vi "Noise Cancel.vi"(9 "Config":T2={"Ref Index"=1, "Active Index"=2, "Gain"=1.1, "Channel name"="Mic Diff", "Enable"=FALSE}, 11 "array":waveform(dbl)[](array[waveform])) -> (1 "Channel names":T1, 3 "waveform out":waveform(dbl))   [LabVIEW 2019]
doc: "This example demonstrates how to acquire a continuous amount of data (Waveform) using the DAQ device's internal clock. It also shows how to synchronize two devices for different device families (E Series, S Series, M Series, X Series, DSA, and SC Express), to simultaneously acquire the data.\n\nFor instructions on how to connect your signals to the DAQ device, refer to your device documentation."
panel:
  # "Noise Cancellation"
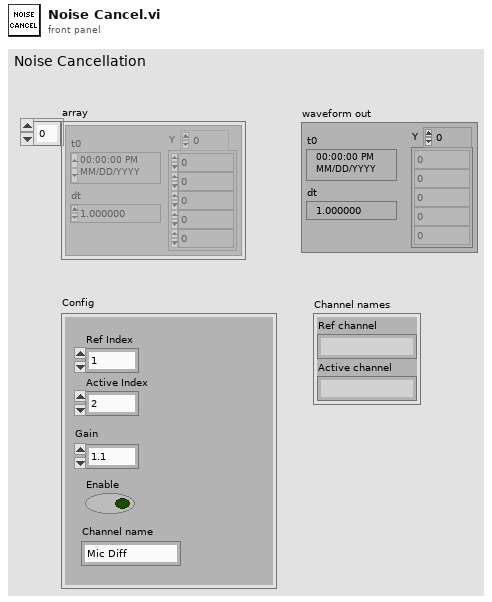
[diagram p1: front panel]
types:
  T1 = cluster{"Ref channel":string, "Active channel":string}
  T2 = cluster{"Ref Index":i32, "Active Index":i32, "Gain":dbl, "Channel name":string, "Enable":bool}
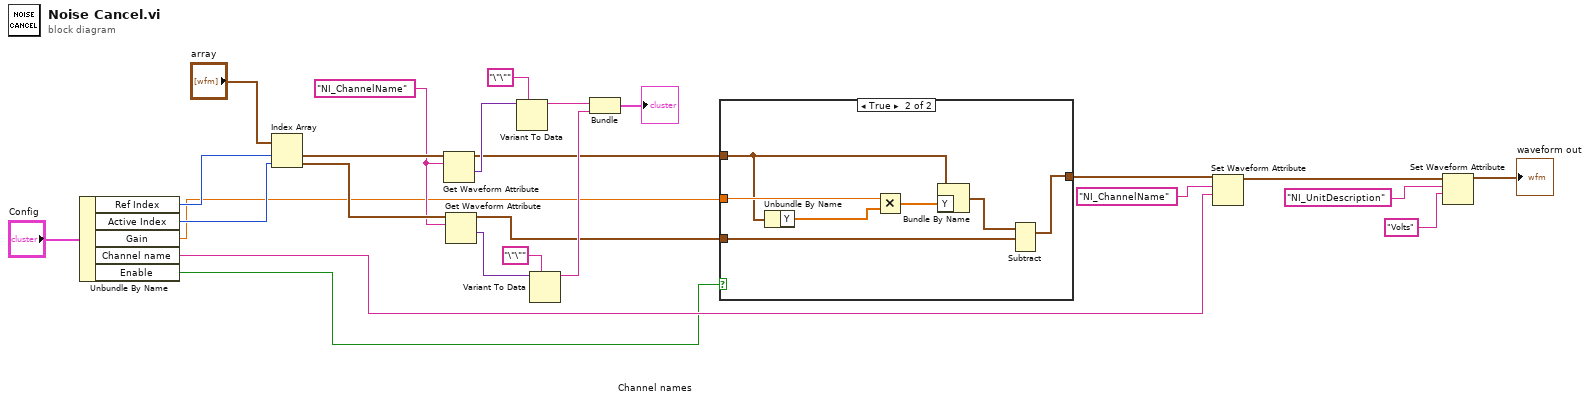
[diagram p0: block diagram]
diagram:
  w18 = "NI_ChannelName" ("name")
  n1 = Unbundle By Name("Config") -> ("Ref Index"=w13:i32, "Active Index"=w12:i32, "Gain"=w4:dbl, "Channel name"=w11:string, "Enable"=w1:bool)
  n2 = Index Array(array="array", index #1=w13, index #2=w12) -> (element #1=w20:waveform(dbl), element #2=w19:waveform(dbl))
  n3 = Get Waveform Attribute(6:w18, 7:w20) -> (1:w9:variant, 3:w2:waveform(dbl))  [unwired: 2 in, 2 out]
  n4 = Get Waveform Attribute(6:w18, 7:w19) -> (1:w15:variant, 3:w5:waveform(dbl))  [unwired: 2 in, 2 out]
  n5 = Variant To Data(type="\"\"" ("name"), Variant=w9) -> (data=w8:string)  [unwired: 1 in, 1 out]
  n6 = Variant To Data(type="\"\"" ("name"), Variant=w15) -> (data=w6:string)  [unwired: 1 in, 1 out]
  n7 = Bundle("name"=w8, "name"=w6) -> (→"Channel names":cluster{"name":string, "name":string})  [unwired: 1 in]
  n8 = case shown="True" w1 {
    tunnel: w5 -> [w26 w30]
    tunnel: w4 -> [_ w29]
    tunnel: [w26 w28] -> w3
    tunnel: w2 -> [_ w27]
    frame False {
    }
    frame True {
      n9 = Unbundle By Name(w27) -> ("Y"=w32:dbl[])
      n10 = Multiply(x=w29, y=w32) -> (x*y=w31:dbl[])
      n11 = Bundle By Name(cluster=w27, "Y"=w31) -> (w33:waveform(dbl))
      n12 = Subtract(1:w30, 2:w33) -> (0:w28:waveform(dbl))  [unwired: 1 in, 1 out]
    }
  }
  n13 = Set Waveform Attribute(5:w11, 6:"NI_ChannelName" ("name"), 7:w3) -> (3:w22:waveform(dbl))  [unwired: 1 in, 2 out]
  n14 = Set Waveform Attribute(5:"Volts" ("name"), 6:"NI_UnitDescription" ("name"), 7:w22) -> (3:→"waveform out":waveform(dbl))  [unwired: 1 in, 2 out]
